vi "InclinometerRawConverterLoop.vi"   [LabVIEW 2016]
uses:
  <vilib>/rvi/Emulation/niFpgaGetClockAttributes.vi
  <vilib>/rvi/Emulation/niFpgaSctlEmulationGetInTimedLoop.vi
  <vilib>/rvi/Emulation/niFpgaEmulationReportErrorSimple.vi
  <vilib>/rvi/Emulation/niFpgaEmulationIsFPGAContextNoSignature.vi
  <vilib>/rvi/errors/niFpgaSetErrorForExecOnDevCompSimple.vi
  <vilib>/rvi/eio/common/nirviEmuReportErrorAndStop.vi
  <vilib>/rvi/DataTransferAndStorage/Container/Common/niFpgaContainerGetUniqueNameForEmu.vi
  <vilib>/rvi/FIFO/Fifo_Resource/nirvififoEmulationSetSize.vi
  <vilib>/rvi/FIFO/Fifo_Resource/nirviFifoEmulationQueueMgr.vi
  <instcachedir>/0/nirviFifoEmulationQueueMgr_E5CAEC123FF24DC58D834DCA3CDAA9B5.lvgen/nirviFifoEmulationQueueMgr_E5CAEC123FF24DC58D834DCA3CDAA9B5_035.vi
  <vilib>/Utility/error.llb/Clear Errors.vi
  <vilib>/rvi/FIFO/Fifo_Resource/nirvififoEmulationCreateLock.vi
  <vilib>/rvi/Emulation/niFpgaProcessEmulError.vi
  <vilib>/rvi/FIFO/Fifo_Resource/nirvififoEmulationObtainLock.vi
  <vilib>/rvi/FIFO/Fifo_Resource/nirvififoEmulationReleaseLock.vi
  <vilib>/rvi/occurrence/nirviWaitOnOccurrenceBase.vi
  <vilib>/rvi/errors/nirviReportUnexpectedCaseInternalError.vi
  <vilib>/rvi/errors/nirviReportUnexpectedCaseInternalError (U32).vi
  <userlib>/_NI FLP Library/FPGA/outsideSCTL/FlpLib Divide Shared Instance 0.vi
  <userlib>/_NI FLP Library/FPGA/outsideSCTL/FlpLib Subtract Shared Instance 0.vi
  <userlib>/_NI FLP Library/FPGA/outsideSCTL/FlpLib Negate Outside SCTL.vi
  <userlib>/_NI FLP Library/FPGA/outsideSCTL/FlpLib Greater Than or Equal Shared Instance 0.vi
  <vilib>/rvi/FIFO/Fifo_Resource/nirvififoEmulationDetermineInputValidOut.vi
  <vilib>/rvi/Emulation/niFpgaCriticalErrorInLSC.vi
  <vilib>/rvi/DataTransferAndStorage/Container/XNode/niFpgaContainer.xnode
  <vilib>/rvi/FIFO/Fifo_Resource/nirvififoEmulationRead.vi
  <vilib>/rvi/FIFO/Fifo_Resource/nirvififoEmulationWrite.vi
types:
  T1 = cluster{"Timestamp":u64, "TxBytes":u64, "RxBytes":u64, "TxFrames":u64, "RxFrames":u64, "RawAngle":i32, "ZenithAngle":sgl}
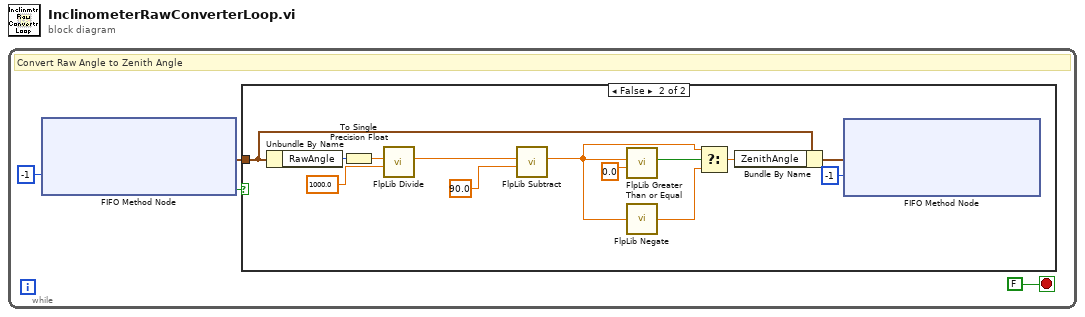
[diagram p0: block diagram]
diagram:
  n1 = while {
    stop <- FALSE stop-if-true
    # "Convert Raw Angle to Zenith Angle"
    n2 = xnode ("FIFO Method Node")("Timeout"=-1) -> ("Element"=w1:T1, "Timed Out?"=w3:bool)  [unwired: 1 in, 1 out]
    n3 = case shown="False" w3 {
      tunnel: w1 -> [_ w16]
      frame True {
      }
      frame False {
        n4 = Unbundle By Name(w16) -> ("RawAngle"=w14:i32)
        n5 = To Single Precision Float(number=w14) -> (single precision float=w13:sgl)
        n6 = call-poly <userlib>:"FlpLib Divide.vi"("y"=sgl 1000.0, "x"=w13) -> ("x/y"=w11:sgl)  [unwired: 5 in]
        n7 = call-poly <userlib>:"FlpLib Subtract.vi"("y"=sgl 90.0, "x"=w11) -> ("x-y"=w7:sgl)  [unwired: 5 in]
        n8 = call-poly <userlib>:"FlpLib Greater Than or Equal.vi"("y"=sgl 0.0, "x"=w7) -> ("x >= y?"=w8:bool)  [unwired: 5 in]
        n9 = call-poly <userlib>:"FlpLib Negate.vi"("x"=w7) -> ("-x"=w6:sgl)  [unwired: 4 in]
        n10 = Select(t=w7, s=w8, f=w6) -> (s? t:f=w5:sgl)
        n11 = Bundle By Name(cluster=w16, "ZenithAngle"=w5) -> (w15:T1)
        n12 = xnode ("FIFO Method Node")("Element"=w15, "Timeout"=-1) -> ()  [unwired: 1 in, 2 out]
      }
    }
  }
